vi "界面示例.vi"() -> ()   [LabVIEW 2010]
panel:
  in  "停止":bool
  in  "信息":string
  out "波形图":dbl[](graph)
  out "油箱":dbl(slide) scale=0.0..10.0
  out "水箱":dbl(slide) scale=0.0..10.0
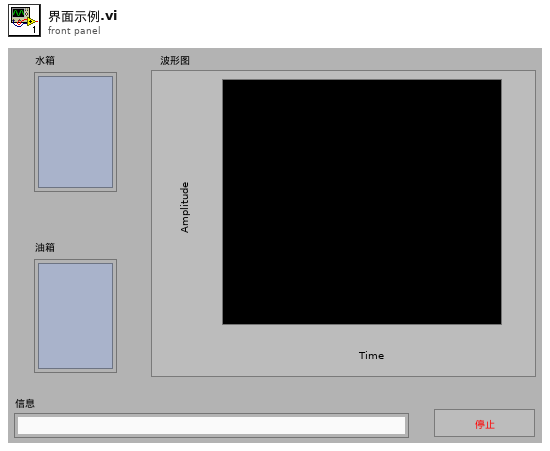
[diagram p1: front panel]
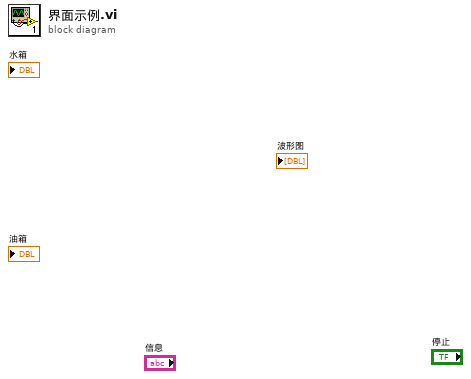
[diagram p0: block diagram]
diagram:
